vi "Read Meta Data (TCP Clst).vi"(6 "options":T3={"ignore timeout error"=TRUE, "timeout ms (1000)"=1000}, 8 "error in":errorcluster, 11 "connection info in":T1) -> (0 "error out":errorcluster, 1 "meta data":T2[](array[typedef]), 3 "connection info out":T1)   [LabVIEW 2010, in "NI STM.lvlib"]
doc: "This VI reads the meta data information from a remote computer. Use this VI to retrieve the variable names and types that a remote computer exports.\n\nThis VI parses the data and returns a cluster containing the meta data information.\n\nCopyright 2015, 2016, 2017 National Instruments Corporation\n\nLicensed under the Apache License, Version 2.0 (the \"License\"); you may not use this file except in compliance with the License.\n\n You may obtain a copy of the License at\n\n http://www.apache.org/licenses/LICENSE-2.0\n\nUnless required by applicable law or agreed to in writing, software distributed under the License is distributed on an \"AS IS\" BASIS, WITHOUT WARRANTIES OR CONDITIONS OF ANY KIND, either express or implied.\n\nSee the License for the specific language governing permissions and limitations under the License."
uses:
  NI STM.lvlib
  SubVIs/MetaDataElement.ctl
  TCP Read Options.ctl
  TCP Connection Info.ctl
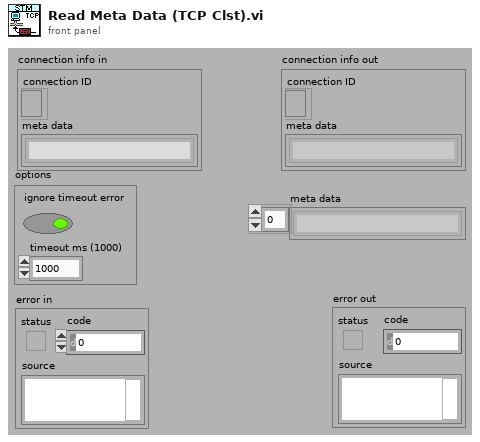
[diagram p1: front panel]
types:
  T1 = typedef "NI STM.lvlib/TCP Connection Info.ctl" = cluster{"connection ID":refnum<k5>, "meta data":T2[]}
  T2 = typedef "NI STM.lvlib/MetaDataElement.ctl" = string
  T3 = typedef "NI STM.lvlib/TCP Read Options.ctl" = cluster{"ignore timeout error":bool, "timeout ms (1000)":i32}
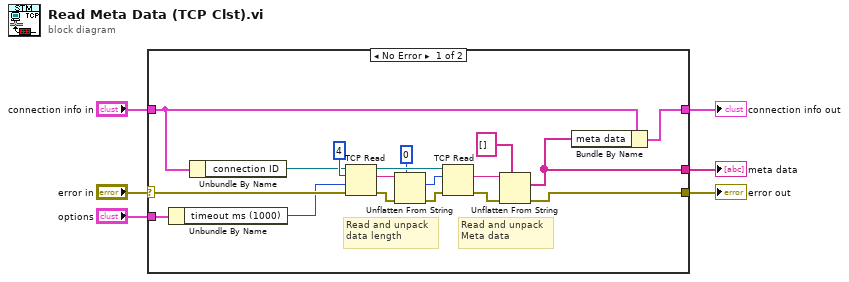
[diagram p0: block diagram]
diagram:
  n1 = case shown="No Error" "error in" {
    selector: "error in" -> [w13 w26]
    tunnel: [w12 _] -> w6
    tunnel: [w24 w26] -> w5
    tunnel: [w11 w25] -> w1
    tunnel: "options" -> [w10 _]
    tunnel: "connection info in" -> [w7 w25]
    frame No Error {
      # "Read and unpack\nMeta data"
      # "Read and unpack\ndata length"
      n2 = Unbundle By Name(w10) -> ("timeout ms (1000)"=w8:i32)
      n3 = Unbundle By Name(w7) -> ("connection ID"=w9:refnum<k5>)
      n4 = TCP Read(connection ID=w9, bytes to read=4, error in (no error)=w13, 9:w8) -> (connection ID out=w21:refnum<k5>, data out=w18:string, error out=w14:errorcluster)  [unwired: 1 out]
      n5 = Unflatten From String(type=0 ("bytes to read"), binary string=w18, error in (no error)=w14) -> (value=w15:i32, error out=w16:errorcluster)  [unwired: 3 out]
      n6 = TCP Read(connection ID=w21, bytes to read=w15, error in (no error)=w16) -> (data out=w20:string, error out=w19:errorcluster)  [unwired: 3 out]
      n7 = Unflatten From String(type=T2[] [] ("Meta data"), binary string=w20, error in (no error)=w19) -> (value=w12:T2[], error out=w24:errorcluster)  [unwired: 3 out]
      n8 = Bundle By Name(cluster=w7, "meta data"=w12) -> (w11:T1)
    }
    frame Error {
    }
  }
  "meta data" <- w6
  "error out" <- w5
  "connection info out" <- w1
